vi "AdjustCorners.vi"(8 "error in":errorcluster, 9 "Map":i8[][](array[numeric]), 10 "Corners":cluster{"Col":i16, "Row":i16}[](array[cluster])) -> (0 "error out":errorcluster, 2 "Corners out":cluster{"Col":i16, "Row":i16}[](array[cluster]))   [LabVIEW 2009, in "Main.lvlib"]
uses:
  Main.lvlib
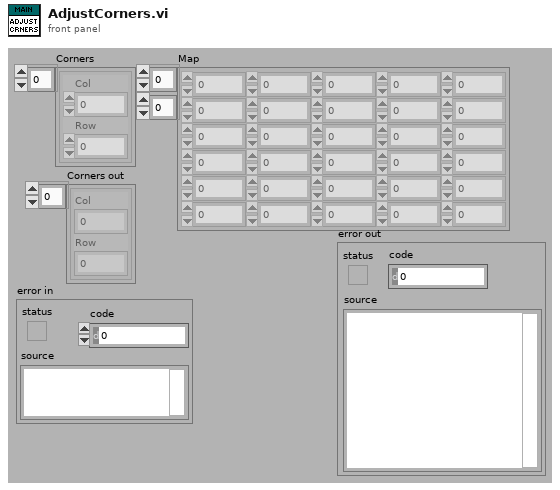
[diagram p1: front panel]
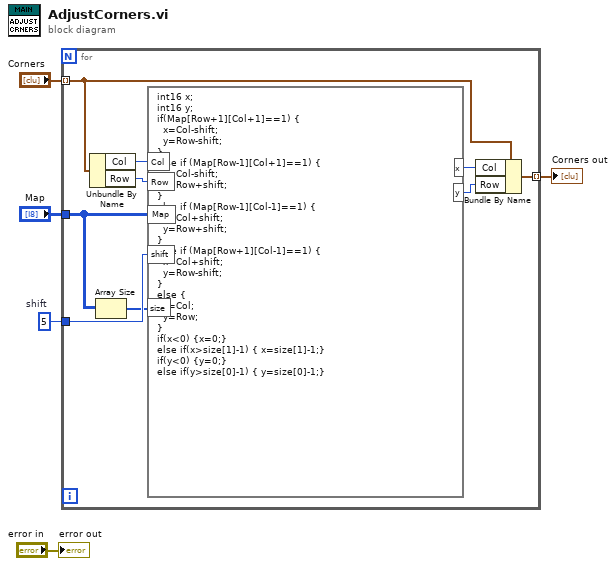
[diagram p0: block diagram]
diagram:
  w3 = i16 5  # shift
  n1 = for {
    tunnel: "Corners" -> [w11] mode=indexing
    tunnel: "Map" -> [w7]
    tunnel: w3 -> [w12]
    tunnel: [w10] -> w2 mode=indexing
    n2 = Unbundle By Name(w11) -> ("Col"=w14:i16, "Row"=w13:i16)
    n3 = Array Size(array=w7) -> (size(s)=w6:i32[])
    n4 = formula code="int16 x;\nint16 y;\nif(Map[Row+1][Col+1]==1) {\n  x=Col-shift;\n  y=Row-shift;\n}\nelse if (Map[Row-1][Col+1]==1) {\n  x=Col-shift;\n  y=Row+shift;\n}\nelse if (Map[Row-1][Col-1]==1) {\n  x=Col+shift;\n  y=Row+shift;\n}\nelse if (Map[Row+1][Col-1]==1) {\n  x=Col+shift;\n  y=Row-shift;\n}\nelse {\n  x=Col;\n  y=Row;\n}\nif(x<0) {x=0;}\nelse if(x>size[1]-1) { x=size[1]-1;}\nif(y<0) {y=0;}\nelse if(y>size[0]-1) { y=size[0]-1;}"("Map"=w7, "Col"=w14, "Row"=w13, "shift"=w12, "size"=w6) -> ("x"=w9:i16, "y"=w8:i16)
    n5 = Bundle By Name(cluster=w11, "Col"=w9, "Row"=w8) -> (w10:cluster{"Col":i16, "Row":i16})
  }
  "Corners out" <- w2
  "error out" <- "error in"
